vi "rosmaster.vi"   [LabVIEW 2015]
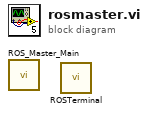
[diagram p0: block diagram]
diagram:
  n1 = call <vilib>:"ROS_Master_Main.vi"() -> ()  [unwired: 4 in]
  n2 = call <vilib>:"ROSTerminal.vi"() -> ()  [unwired: 2 in]
